vi "set_PID.vi"(0 "heat_board_control in":refnum<class "heat_board_control.lvclass">, 5 "P":dbl, 7 "I":dbl, 9 "D":dbl, 11 "error in (no error)":errorcluster) -> (4 "heat_board_control out":refnum<class "heat_board_control.lvclass">, 15 "error out":errorcluster)   [LabVIEW 2015, in "heat_board_control.lvclass"]
uses:
  heat_board_control.lvclass
  heat_board_control.lvclass/heat_board_control.ctl
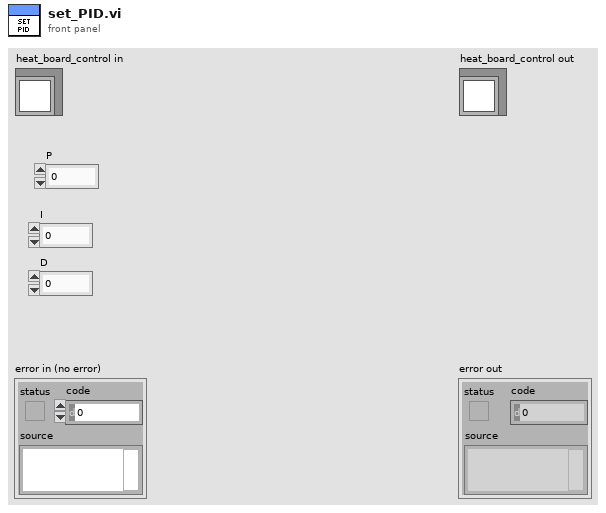
[diagram p1: front panel]
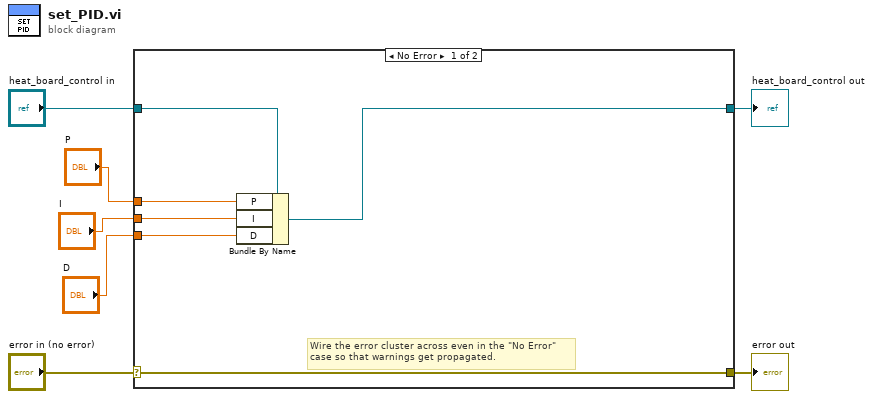
[diagram p0: block diagram]
diagram:
  n1 = case shown="No Error" "error in (no error)" {
    selector: "error in (no error)" -> [w13 w15]
    tunnel: [w13 w15] -> w6
    tunnel: [w8 w14] -> w4
    tunnel: "heat_board_control in" -> [w9 w14]
    tunnel: "P" -> [w12 _]
    tunnel: "I" -> [w11 _]
    tunnel: "D" -> [w10 _]
    frame No Error {
      # "Wire the error cluster across even in the \"No Error\"\ncase so that warnings get propagated."
      n2 = Bundle By Name(cluster=w9, "P"=w12, "I"=w11, "D"=w10) -> (w8:refnum<class "heat_board_control.lvclass">)
    }
    frame Error {
    }
  }
  "error out" <- w6
  "heat_board_control out" <- w4
